vi "GCD of P(x) and Q(x).vi"   [LabVIEW 2024, in "NI_AALPro.lvlib"]
doc: "<p>Computes the greatest common divisor for two polynomials <strong>P(x)</strong> and <strong>Q(x)</strong> with the <strong>tolerance</strong> you specify. The data types you wire to the <strong>P(x)</strong> and <strong>Q(x)</strong> inputs determine the polymorphic instance to use.</p>"
uses:
  NI_AALPro.lvlib
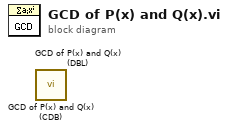
[diagram p0: block diagram]
diagram:
  n1 = call "GCD of P(x) and Q(x) (CDB).vi"() -> ()  [unwired: 10 in, 2 out]
  n2 = call "GCD of P(x) and Q(x) (DBL).vi"() -> ()  [unwired: 10 in, 2 out]
